vi "Trigger Timestamp.vi"(8 "error in (no error)":errorcluster, 11 "TrialBasedExperiment in":refnum<class "TrialBasedExperiment.lvclass">) -> (0 "error out":errorcluster, 3 "TrialBasedExperiment out":refnum<class "TrialBasedExperiment.lvclass">)   [LabVIEW 2010, in "TrialBasedExperiment.lvclass"]
uses:
  TrialBasedExperiment.lvclass
  <vilib>/DAQmx/write.llb/DAQmx Write (Digital Bool 1Line 1Point).vi
  <vilib>/DAQmx/create/channels.llb/DAQmx Create Channel (DO-Digital Output).vi
  <vilib>/daqmx/miscellaneous.llb/DAQmx Fill In Error Info.vi
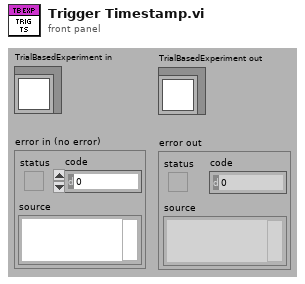
[diagram p1: front panel]
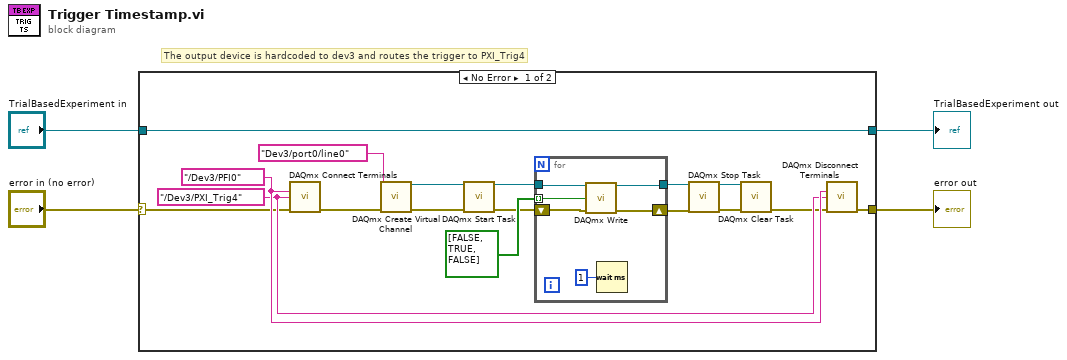
[diagram p0: block diagram]
diagram:
  # "The output device is hardcoded to dev3 and routes the trigger to PXI_Trig4"
  n1 = case shown="No Error" "error in (no error)" {
    selector: "error in (no error)" -> [w11 w29]
    tunnel: [w9 w29] -> w3
    tunnel: [w21 w28] -> w1
    tunnel: "TrialBasedExperiment in" -> [w21 w28]
    frame No Error {
      w12 = tag "/Dev3/PXI_Trig4" ("destination terminal")
      w13 = tag "/Dev3/PFI0" ("source terminal")
      n2 = call <vilib>:"DAQmx Connect Terminals.vi"("source terminal"=w13, "destination terminal"=w12, "error in"=w11) -> ("error out"=w6:errorcluster)  [unwired: 12 in]
      n3 = call-poly <vilib>:"DAQmx Create Virtual Channel.vi"("lines"=tag "Dev3/port0/line0", "error in"=w6) -> ("task out"=w5:refnum<k21>, "error out"=w7:errorcluster)  [unwired: 12 in]
      n4 = call <vilib>:"DAQmx Start Task.vi"("task/channels in"=w5, "error in"=w7) -> ("task out"=w17:refnum<k21>, "error out"=w15:errorcluster)  [unwired: 12 out]
      n5 = for {
        tunnel: bool[] [FALSE, TRUE, FALSE] -> [w27] mode=indexing
        tunnel: w17 -> [w26]
        tunnel: [w25] -> w16
        shift-right: [w22] -> w14
        shift-left: w15 -> [w23]
        n6 = call-poly <vilib>:"DAQmx Write.vi"("task/channels in"=w26, "data"=w27, "error in"=w23) -> ("task out"=w25:refnum<k21>, "error out"=w22:errorcluster)  [unwired: 1 in, 10 out]
        n7 = Wait (ms)(milliseconds to wait=u32 1) -> ()  [unwired: 1 out]
      }
      n8 = call <vilib>:"DAQmx Stop Task.vi"("task/channels in"=w16, "error in"=w14) -> ("task out"=w20:refnum<k21>, "error out"=w19:errorcluster)  [unwired: 12 out]
      n9 = call <vilib>:"DAQmx Clear Task.vi"("task in"=w20, "error in"=w19) -> ("error out"=w10:errorcluster)  [unwired: 13 out]
      n10 = call <vilib>:"DAQmx Disconnect Terminals.vi"("source terminal"=w13, "destination terminal"=w12, "error in"=w10) -> ("error out"=w9:errorcluster)  [unwired: 12 in]
    }
    frame Error {
    }
  }
  "error out" <- w3
  "TrialBasedExperiment out" <- w1
